vi "Get Desired Size.vi"(8 "error in (no error)":errorcluster, 11 "WebProjectPanel in":refnum<class "WebProjectPanel.lvclass">) -> (0 "error out":errorcluster, 2 "Desired Size":T1, 3 "WebProjectPanel out":refnum<class "WebProjectPanel.lvclass">)   [LabVIEW 2020, in "PicoG-Processor.lvlib" / "WebProjectPanel.lvclass"]
uses:
  WebProjectPanel.lvclass
  <vilib>/IlluminatedG/IG OOPanel/OOPanel/ArrayPanel/Desired Size.ctl
  <vilib>/IlluminatedG/IG OOPanel/OOPanel/ArrayPanel/ArrayPanel.lvclass
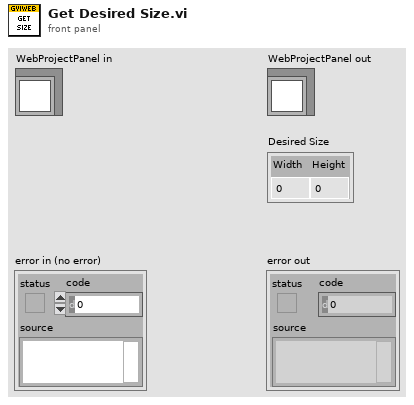
[diagram p1: front panel]
types:
  T1 = typedef "OOPanel.lvlib/ArrayPanel.lvclass/Desired Size.ctl" = cluster{"Width":u32, "Height":u32}
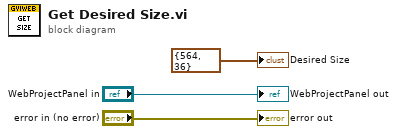
[diagram p0: block diagram]
diagram:
  "error out" <- "error in (no error)"
  "WebProjectPanel out" <- "WebProjectPanel in"
  "Desired Size" <- T1 {"Width"=564, "Height"=36} ("Desired Size")
